vi "CheckForOriginator.vi"(8 "error in (no error)":errorcluster, 11 "data in":T1) -> (0 "error out":errorcluster, 1 "group":string, 2 "originator":string, 3 "found":bool)   [LabVIEW 2017, in "DataFlow.lvlib"]
uses:
  <vilib>/addons/InsightCM/Devices/Shared/Common/DataFlow/DataFlow.lvlib
  <vilib>/addons/InsightCM/Devices/Shared/Common/DataFlow/controls/Data.ctl
  <vilib>/addons/InsightCM/Utilities/DataAccessors/controls/wfmSGL_DVR.ctl
  <vilib>/addons/PointValueMap/controls/PointMap.ctl
  <vilib>/addons/InsightCM/Devices/Shared/Common/DataFlow/controls/Type.ctl
  <vilib>/addons/PointValueMap/subVIs/Point_Read_string.vi
  <vilib>/addons/PointValueMap/PointValueMap.lvlib
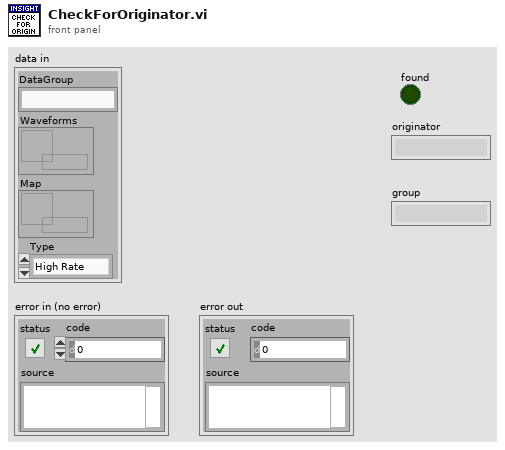
[diagram p1: front panel]
types:
  T1 = typedef "DataFlow.lvlib/Data.ctl" = cluster{"DataGroup":string, "Waveforms":T2, "Map":T3, "Type":T4}
  T2 = typedef "wfmSGL_DVR.ctl" = refnum<data-value>
  T3 = typedef "PointValueMap.lvlib/PointMap.ctl" = refnum<data-value>
  T4 = typedef "DataFlow.lvlib/Type.ctl" = enum16{"High Rate", "Low Rate", "Burst Mode"}
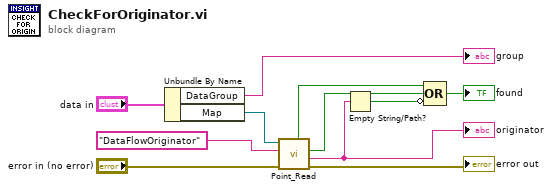
[diagram p0: block diagram]
diagram:
  n1 = Unbundle By Name("data in") -> ("DataGroup"=→"group":string, "Map"=w10:T3)
  n2 = call-poly <vilib>:"Point_Read.vi"("Error In"="error in (no error)", "Tag"="DataFlowOriginator", "Map"=w10) -> ("Error Out"=→"error out":errorcluster, "Value"=w5:string, "Found?"=w7:bool, "Valid?"=w6:bool)  [unwired: 3 in, 2 out]
  "originator" <- w5
  n3 = Empty String/Path?(string/path=w5) -> (empty?=w4:bool)
  n4 = Compound Arithmetic op=OR(w6, w7, invert w4) -> (→"found":bool)
